vi "Мультиплексор.vi"(1 "?":bool, 2 "2":bool, 3 "1":bool) -> (0 "?":bool)   [LabVIEW 2017]
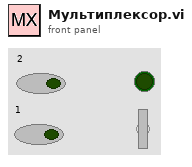
[diagram p1: front panel]
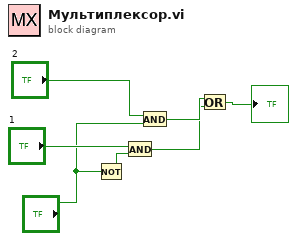
[diagram p0: block diagram]
diagram:
  n1 = Not(x="?") -> (.not. x?=w5:bool)
  n2 = And(x="1", y=w5) -> (x .and. y?=w2:bool)
  n3 = And(x="2", y="?") -> (x .and. y?=w3:bool)
  n4 = Or(x=w3, y=w2) -> (x .or. y?=→"?":bool)
